vi "Actor Core.vi"(8 "error in":errorcluster, 11 "Synchronization in":refnum<class "Synchronization.lvclass">) -> (0 "error out":errorcluster, 3 "Actor out":refnum<class "Actor.lvclass">)   [LabVIEW 2015, in "Synchronization Actor.lvlib" / "Synchronization.lvclass"]
doc: "(<B>Filename</B>: Actor Framework.lvlib:Actor.lvclass:Actor Core.vi)\n\nReceives messages to the actor, reacts to them, and initiates any error handling that may shut the actor down.\n\nDescendant classes may override this VI to append parallel tasks for the actor to complete while it handles messages. Overrides use the Call Parent Method node."
uses:
  Synchronization.lvclass
  <vilib>/ActorFramework/Actor/Actor.lvclass
  Controls/LED Bar.ctl
  Synchronization.lvclass/Synchronization.ctl
  SCADA Core/SCADA Abstract Messages/Simple Command Status Msg/Simple Command Status.ctl
  IED Actor/IED/Controls/Generation Mode.ctl
  <vilib>/ActorFramework/Message Enqueuer/Message Priority.ctl
  <vilib>/ActorFramework/Actor/Actor.lvclass/Actor.ctl
  IED Actor/IED Messages/Set Generation Mode Msg/Set Generation Mode Msg.lvclass/Set Generation Mode Msg.ctl
  <vilib>/ActorFramework/Message Enqueuer/Message Enqueuer.lvclass/Message Enqueuer.ctl
  IED Actor/IED Messages/Island Watch Msg/Island Watch Msg.lvclass/Island Watch Msg.ctl
  SCADA Core/SCADA Response Messages/Return Synchronize Status Msg/Return Synchronize Status Msg.lvclass/Return Synchronize Status Msg.ctl
  <vilib>/ActorFramework/Message Enqueuer/Enqueue.vi
  <vilib>/ActorFramework/Message Enqueuer/Init from Existing Queue.vi
  <vilib>/ActorFramework/Message Priority Queue/Priority Enqueue.vi
  <vilib>/Modbus/master/Modbus Master.lvclass
  IED Actor/IED Messages/Set Generation Mode Msg/Set Generation Mode Msg.lvclass
  IED Actor/IED Messages/Island Watch Msg/Island Watch Msg.lvclass
  <vilib>/ActorFramework/Message Enqueuer/Message Enqueuer.lvclass
  SCADA Core/SCADA Response Messages/Return Synchronize Status Msg/Return Synchronize Status Msg.lvclass
  <vilib>/ActorFramework/Stop Msg/Stop Msg.lvclass
  SCADA Core/SCADA Abstract Messages/Simple Command Status Msg/Simple Command Status Msg.lvclass
  IED Actor/IED/IED.lvclass
panel:
  out "LED Bar":T1
  # "Synchronizing"
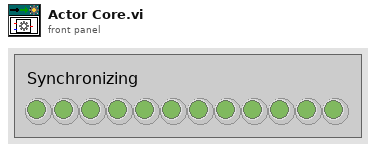
[diagram p1: front panel]
types:
  T1 = typedef "Synchronization Actor.lvlib/Synchronization.lvclass/LED Bar.ctl" = bool[]
  T2 = typedef "SCADA Core.lvlib/Simple Command Status Msg.lvclass/Simple Command Status.ctl" = enum16{"Success", "Failure"}
  T3 = typedef "Actor Framework.lvlib/Message Enqueuer.lvclass/Message Priority.ctl" = enum16{"Low", "Normal", "High"}
  T4 = typedef "IED Actor.lvlib/IED.lvclass/Generation Mode.ctl" = enum16{"P/Q", "V/f"}
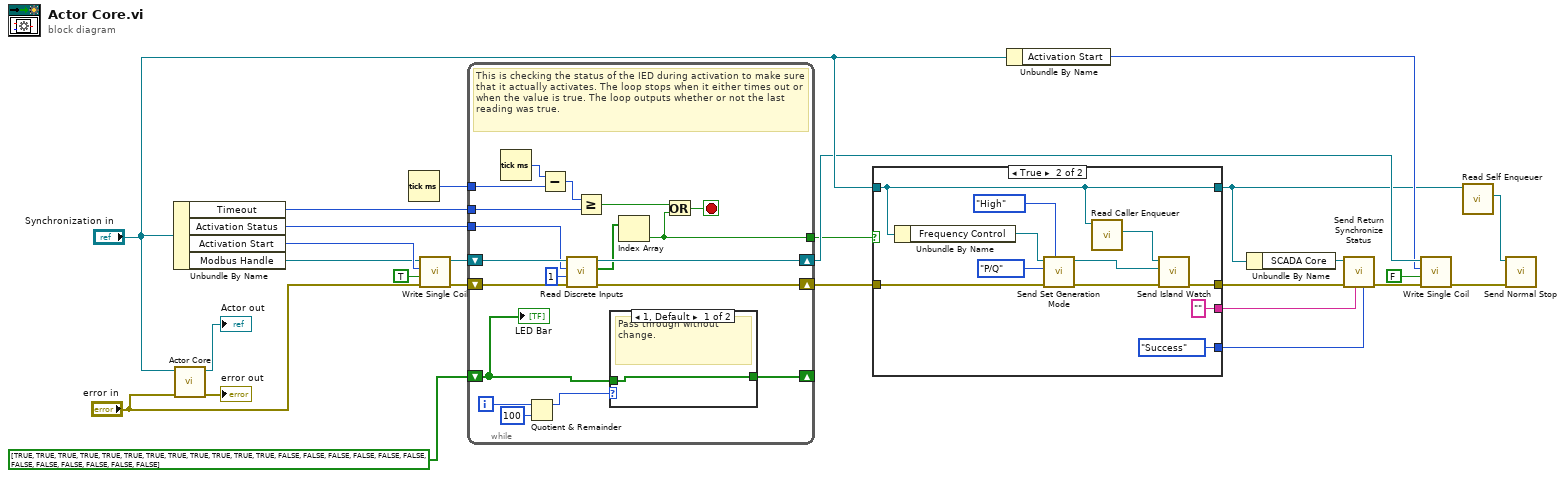
[diagram p0: block diagram]
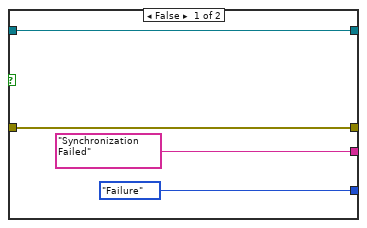
[diagram p2: hidden frame]
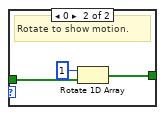
[diagram p3: hidden frame]
diagram:
  n1 = Unbundle By Name("Synchronization in") -> ("Timeout"=w17:u32, "Activation Status"=w18:u16, "Activation Start"=w22:u16, "Modbus Handle"=w2:refnum<class "Modbus Master.lvclass">)
  n2 = call-parent "Actor Core.vi"("error in"="error in", "Actor in"="Synchronization in") -> ("error out"=→"error out":errorcluster, "Actor out"=→"Actor out":refnum<class "Actor.lvclass">)  [unwired: 8 in]
  n3 = Tick Count (ms)() -> (millisecond timer value=w23:u32)
  n4 = call-dynamic "Write Single Coil.vi"("error in (no error)"="error in", "coil value"=TRUE, "address"=w22, "Modbus master in"=w2) -> ("error out"=w19:errorcluster, "Modbus master out"=w20:refnum<class "Modbus Master.lvclass">)  [unwired: 6 in]
  n5 = while {
    tunnel: w23 -> [w44]
    tunnel: w17 -> [w42]
    tunnel: w18 -> [w38]
    shift-right: [w32] -> w11
    shift-left: w19 -> [w37]
    tunnel: [w33] -> w13
    shift-right: [w35] -> w16
    shift-left: w20 -> [w39]
    shift-right: [w30] -> _
    shift-left: bool[] [TRUE, TRUE, TRUE, TRUE, TRUE, TRUE, TRUE, TRUE, TRUE, TRUE, TRUE, TRUE, FALSE, FALSE, FALSE, FALSE, FALSE, FALSE, FALSE, FALSE, FALSE, FALSE, FALSE, FALSE] -> [w31]
    i -> [w29]
    stop <- w40 stop-if-true
    # "This is checking the status of the IED during activation to make sure that it actually activates. The loop stops when it either times out or when the value is true. The loop outputs whether or not the last reading was true."
    n6 = Tick Count (ms)() -> (millisecond timer value=w45:u32)
    n7 = Quotient & Remainder(x=w29, y=100) -> (x-y*floor(x/y)=w27:i32)  [unwired: 1 out]
    n8 = Subtract(x=w45, y=w44) -> (x-y=w43:u32)
    n9 = call-dynamic "Read Discrete Inputs.vi"("error in (no error)"=w37, "number of discrete inputs"=u16 1 ("number of coils"), "starting address"=w38, "Modbus master in"=w39) -> ("error out"=w32:errorcluster, "discrete input values"=w34:bool[], "Modbus master out"=w35:refnum<class "Modbus Master.lvclass">)  [unwired: 5 in]
    n10 = Greater Or Equal?(x=w43, y=w42) -> (x >= y?=w41:bool)
    n11 = case shown="1, Default" w27 {
      tunnel: w31 -> [w46 w49]
      tunnel: [w46 w47] -> w30
      frame 1, Default {
        # "Pass through without change."
      }
      frame 0 {
        # "Rotate to show motion."
        n12 = Rotate 1D Array(1:w49, 2:1 ("n")) -> (0:w47:bool[])
      }
    }
    n13 = Index Array(array=w34) -> (element=w33:bool)  [unwired: 1 in]
    n14 = Or(x=w41, y=w33) -> (x .or. y?=w40:bool)
    "LED Bar" <- w31
  }
  n15 = case shown="True" w13 {
    tunnel: w11 -> [w52 w64]
    tunnel: "Synchronization in" -> [w53 w58]
    tunnel: [w52 w56] -> w10
    tunnel: [w53 w58] -> w8
    tunnel: ["Synchronization Failed" ("error") "" ("error")] -> w6
    tunnel: [Simple_Command_Status."Failure" ("Status") Simple_Command_Status."Success" ("Status")] -> w5
    frame False {
    }
    frame True {
      n16 = Unbundle By Name(w58) -> ("Frequency Control"=w61:refnum<class "Message Enqueuer.lvclass">)
      n17 = call "Send Set Generation Mode.vi"("Message Priority (Normal)"=Message_Priority."High", "error in (no error)"=w64, "Mode"=Generation_Mode."P/Q", "Message Enqueuer"=w61) -> ("error out"=w57:errorcluster, "Message Enqueuer out"=w54:refnum<class "Message Enqueuer.lvclass">)  [unwired: 6 in]
      n18 = call <vilib>:"Read Caller Enqueuer.vi"("Actor"=w58) -> ("Caller Enqueuer"=w55:refnum<class "Message Enqueuer.lvclass">)  [unwired: 10 in]
      n19 = call "Send Island Watch.vi"("error in (no error)"=w57, "Frequency Control"=w54, "Message Enqueuer"=w55) -> ("error out"=w56:errorcluster)  [unwired: 7 in, 1 out]
    }
  }
  n20 = Unbundle By Name("Synchronization in") -> ("Activation Start"=w15:u16)
  n21 = Unbundle By Name(w8) -> ("SCADA Core"=w7:refnum<class "Message Enqueuer.lvclass">)
  n22 = call "Send Return Synchronize Status.vi"("Status"=w5, "error"=w6, "error in (no error)"=w10, "Message Enqueuer"=w7) -> ("error out"=w9:errorcluster)  [unwired: 6 in, 1 out]
  n23 = call-dynamic "Write Single Coil.vi"("error in (no error)"=w9, "coil value"=FALSE, "address"=w15, "Modbus master in"=w16) -> ("error out"=w4:errorcluster)  [unwired: 6 in, 1 out]
  n24 = call <vilib>:"Read Self Enqueuer.vi"("Actor"=w8) -> ("Self Enqueuer"=w12:refnum<class "Message Enqueuer.lvclass">)  [unwired: 10 in]
  n25 = call <vilib>:"Send Normal Stop.vi"("error in (no error)"=w4, "Message Enqueuer"=w12) -> ()  [unwired: 9 in, 1 out]
